vi "DT_yadcf_GetDependencyFiles.vi"() -> (1 "rel. Filepaths .js":path[](array[path]), 2 "rel. Filepaths .css":path[](array[path]))   [LabVIEW 2014]
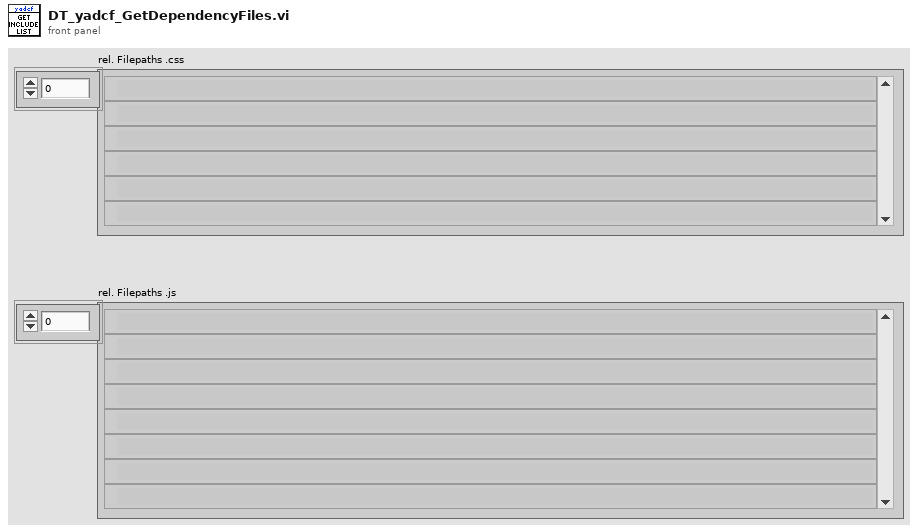
[diagram p1: front panel]
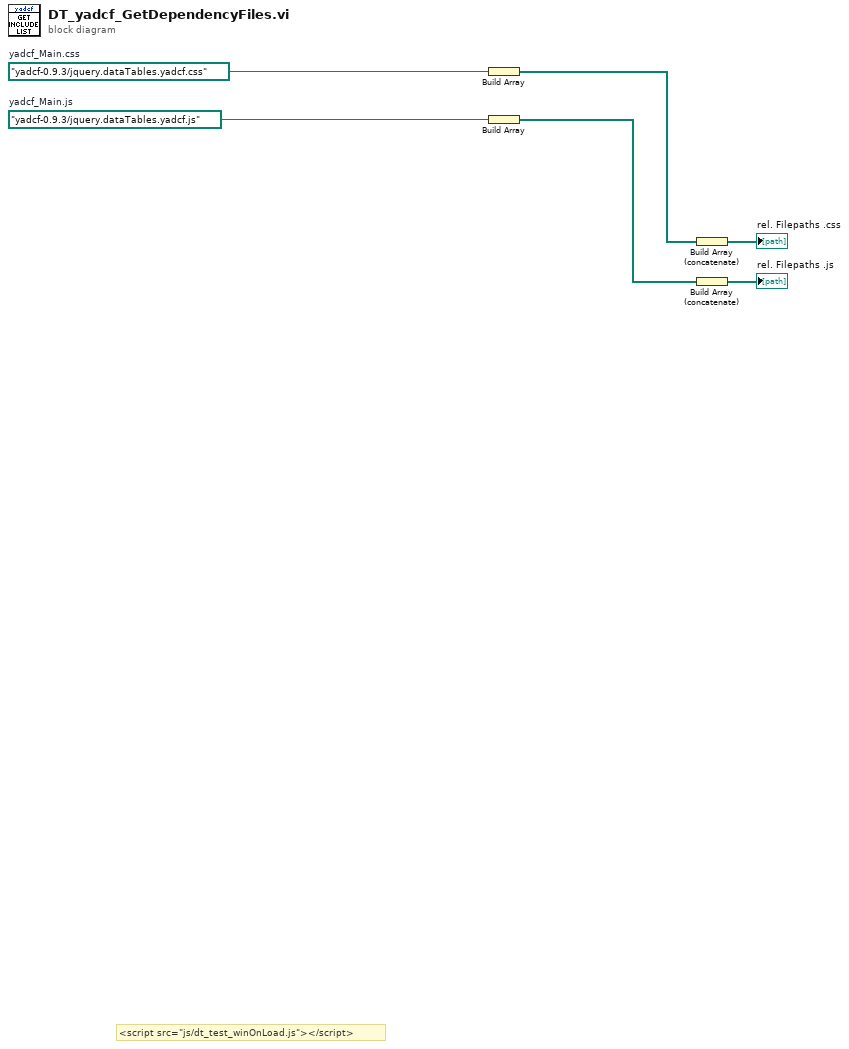
[diagram p0: block diagram]
diagram:
  w2 = path "yadcf-0.9.3/jquery.dataTables.yadcf.js"  # yadcf_Main.js
  w6 = path "yadcf-0.9.3/jquery.dataTables.yadcf.css"  # yadcf_Main.css
  # "<script src=\"js/dt_test_winOnLoad.js\"></script>"
  n1 = Build Array(w6) -> (w5:path[])
  n2 = Build Array(w2) -> (w1:path[])
  n3 = Build Array (concatenate)(w5) -> (→"rel. Filepaths .css":path[])
  n4 = Build Array (concatenate)(w1) -> (→"rel. Filepaths .js":path[])
